vi "Get stack name.vi"(0 "Module?":bool, 1 "Baseplate Type":string, 5 "Protoname (baselayer)":string="320-PH-F2CX-CM-0055", 7 "Sensor thickness":string, 9 "Geometry":string="XX-", 11 "Resolution":string="HD", 14 "Hexaboard ROC version":string="X") -> (8 "Stack name":string="320-PH-F1-CM-0054")   [LabVIEW 2021, in "Stack.lvclass"]
uses:
  Stack.lvclass
  <vilib>/JDP Science/JDP Science Common Utilities/JDP Utility.lvlib
panel:
  out "Institution":string="CM"
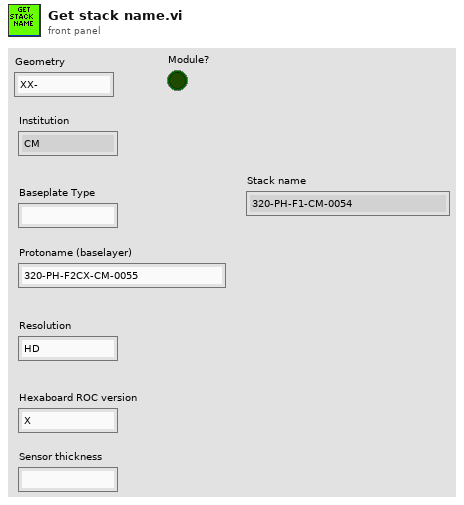
[diagram p1: front panel]
types:
  T1 = typedef "File Paths.ctl" = cluster{"Glue Pattern Folder":path, "Carrier Tray Folder":path, "Pick Up Tool Fixture Folder":path, "Components Folder":path, "Bellows Tool Offset.txt":path, "Pick Up Tool Offset.txt":path, "Dispense Tip Offset.txt":path, "Log Files":path, "Gantry Assembly Map.txt":path, "Syringe and offset map.txt":path, "Controllers Folder":path, "Local dbase config":path}
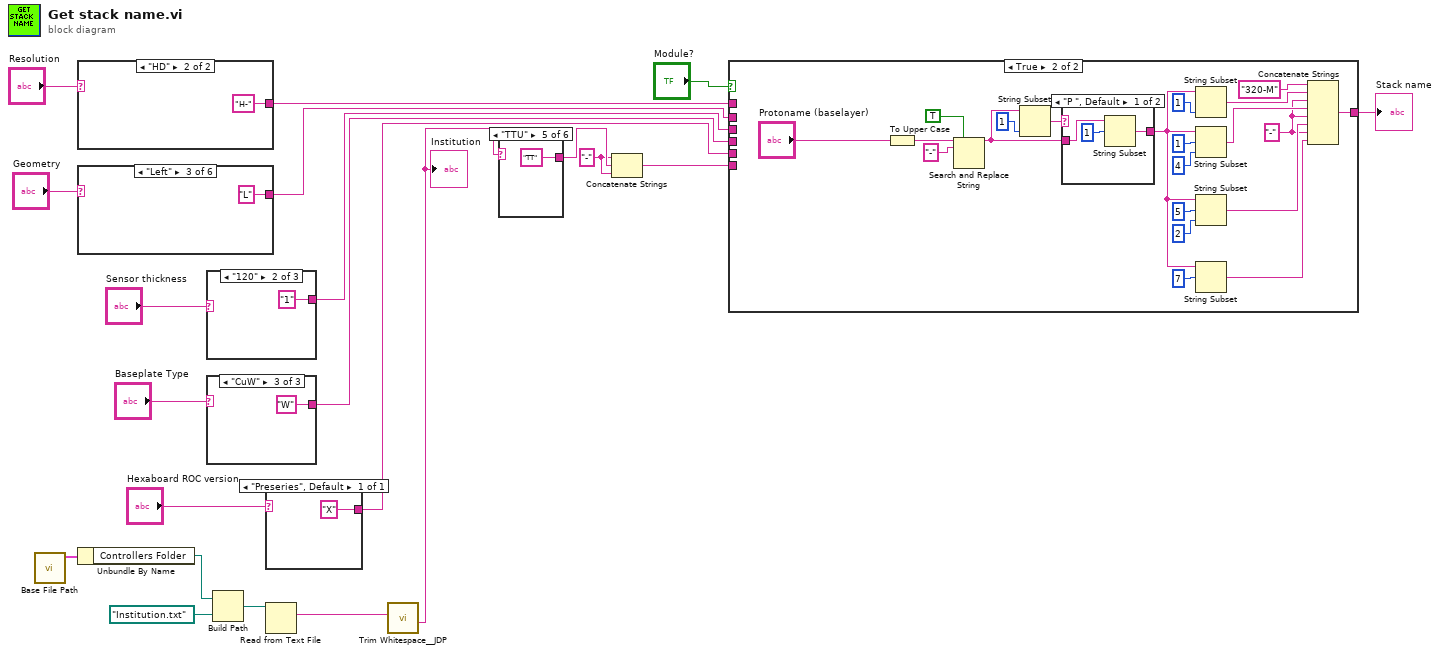
[diagram p0: block diagram]
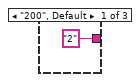
[diagram p2: hidden frame]
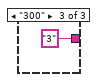
[diagram p3: hidden frame]
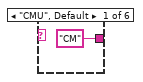
[diagram p4: hidden frame]
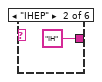
[diagram p5: hidden frame]
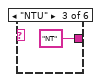
[diagram p6: hidden frame]
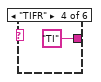
[diagram p7: hidden frame]
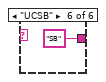
[diagram p8: hidden frame]
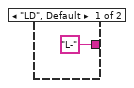
[diagram p9: hidden frame]
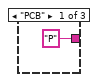
[diagram p10: hidden frame]
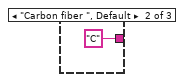
[diagram p11: hidden frame]
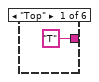
[diagram p12: hidden frame]
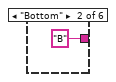
[diagram p13: hidden frame]
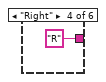
[diagram p14: hidden frame]
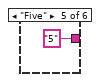
[diagram p15: hidden frame]
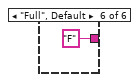
[diagram p16: hidden frame]
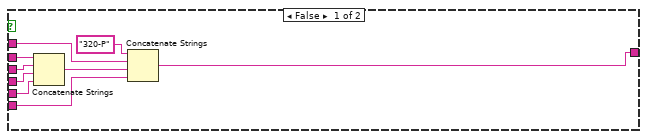
[diagram p17: hidden frame]
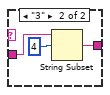
[diagram p18: hidden frame]
diagram:
  w1 = "-" ("string")
  n1 = call "Base File Path.vi"() -> ("Paths Out"=w9:T1)  [unwired: 11 in]
  n2 = case shown="\"HD\"" "Resolution" {
    tunnel: ["L-" "H-"] -> w14
    frame "LD", Default {
    }
    frame "HD" {
    }
  }
  n3 = case shown="\"Left\"" "Geometry" {
    tunnel: ["T" "B" "L" "R" "5" "F"] -> w17
    frame "Top" {
    }
    frame "Bottom" {
    }
    frame "Left" {
    }
    frame "Right" {
    }
    frame "Five" {
    }
    frame "Full", Default {
    }
  }
  n4 = Unbundle By Name(w9) -> ("Controllers Folder"=w8:path)
  n5 = case shown="\"120\"" "Sensor thickness" {
    tunnel: ["2" "1" "3"] -> w2
    frame "200", Default {
    }
    frame "120" {
    }
    frame "300" {
    }
  }
  n6 = case shown="\"CuW\"" "Baseplate Type" {
    tunnel: ["P" "C" "W"] -> w12
    frame "PCB" {
    }
    frame "Carbon fiber ", Default {
    }
    frame "CuW" {
    }
  }
  n7 = Build Path(base path=w8, name or relative path=path "Institution.txt") -> (appended path=w6:path)
  n8 = case shown="\"Preseries\", Default" "Hexaboard ROC version" {
    tunnel: ["X"] -> w11
    frame "Preseries", Default {
    }
  }
  n9 = Read from Text File(file (use dialog)=w6) -> (text=w5:string)  [unwired: 3 in, 3 out]
  n10 = call <vilib>:"Trim Whitespace__JDP.vi"("String in"=w5) -> ("String out"=w4:string)  [unwired: 6 in]
  "Institution" <- w4
  n11 = case shown="\"TTU\"" w4 {
    tunnel: ["CM" "IH" "NT" "TI" "TT" "SB"] -> w10
    frame "CMU", Default {
    }
    frame "IHEP" {
    }
    frame "NTU" {
    }
    frame "TIFR" {
    }
    frame "TTU" {
    }
    frame "UCSB" {
    }
  }
  n12 = Concatenate Strings(w1, w10, w1) -> (w20:string)
  n13 = case shown="True" "Module?" {
    tunnel: [w45 w54] -> w19
    tunnel: w20 -> [w50 _]
    tunnel: w17 -> [w49 _]
    tunnel: w14 -> [w43 _]
    tunnel: w2 -> [w51 _]
    tunnel: w12 -> [w47 _]
    tunnel: w11 -> [w46 _]
    frame False {
      n14 = Concatenate Strings(w49, w51, w47, w46) -> (w48:string)
      n15 = Concatenate Strings("320-P" ("string"), w43, w48, w50) -> (w45:string)
    }
    frame True {
      w61 = "-" ("string")
      n16 = To Upper Case(1:"Protoname (baselayer)") -> (0:w52:string)
      n17 = Search and Replace String(replace all?=TRUE ("replace all? (F)"), input string=w52, search string="-") -> (result string=w68:string)  [unwired: 5 in, 3 out]
      n18 = String Subset(string=w68, length (rest)=1 ("length (rest)")) -> (substring=w69:string)  [unwired: 1 in]
      n19 = case shown="\"P \", Default" w69 {
        tunnel: w68 -> [w75 w78]
        tunnel: [w73 w77] -> w66
        frame "P ", Default {
          n20 = String Subset(string=w75, offset (0)=1 ("length (rest)")) -> (substring=w73:string)  [unwired: 1 in]
        }
        frame "3" {
          n21 = String Subset(string=w78, offset (0)=4) -> (substring=w77:string)  [unwired: 1 in]
        }
      }
      n22 = String Subset(string=w66, length (rest)=1 ("length (rest)")) -> (substring=w65:string)  [unwired: 1 in]
      n23 = String Subset(string=w66, offset (0)=1, length (rest)=4 ("length (rest)")) -> (substring=w64:string)
      n24 = String Subset(string=w66, offset (0)=5, length (rest)=2 ("length (rest)")) -> (substring=w63:string)
      n25 = String Subset(string=w66, offset (0)=7) -> (substring=w62:string)  [unwired: 1 in]
      n26 = Concatenate Strings("320-M" ("string"), w65, w61, w64, w61, w63, w61, w62) -> (w54:string)
    }
  }
  "Stack name" <- w19
